vi "MCLB_IndexArray_Tests.vi"(11 "error in":errorcluster) -> (15 "error out":errorcluster)   [LabVIEW 2016, in "DronaTest.lvlib"]
uses:
  DronaTest.lvlib
  APIs/Stimulus/ControlValue/SetValueAuto.vi
  APIs/Stimulus/ControlValue/Controls/MC Listbox/SetValueByArrayIndex.vi
  APIs/Assert/AssertControlValue/Equal.vi
  <vilib>/addons/_JKI Toolkits/Caraya/classes/Assert/Assert Error.vi
  <vilib>/addons/_JKI Toolkits/Caraya/classes/Test/Test.lvclass
  Drona.lvlib
  <vilib>/SLL Toolkit/SLL Debug/SLL Debug.lvlib
  APIs/Stimulus/ControlValue/ControlValue.lvlib
  APIs/Assert/AssertControlValue/AssertControlValue.lvlib
  <vilib>/addons/_JKI Toolkits/Caraya/classes/Assert/Assert.lvclass
  APIs/Stimulus/ControlValue/Controls/MC Listbox/StimulusMCListbox.lvlib
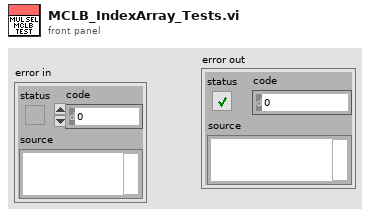
[diagram p1: front panel]
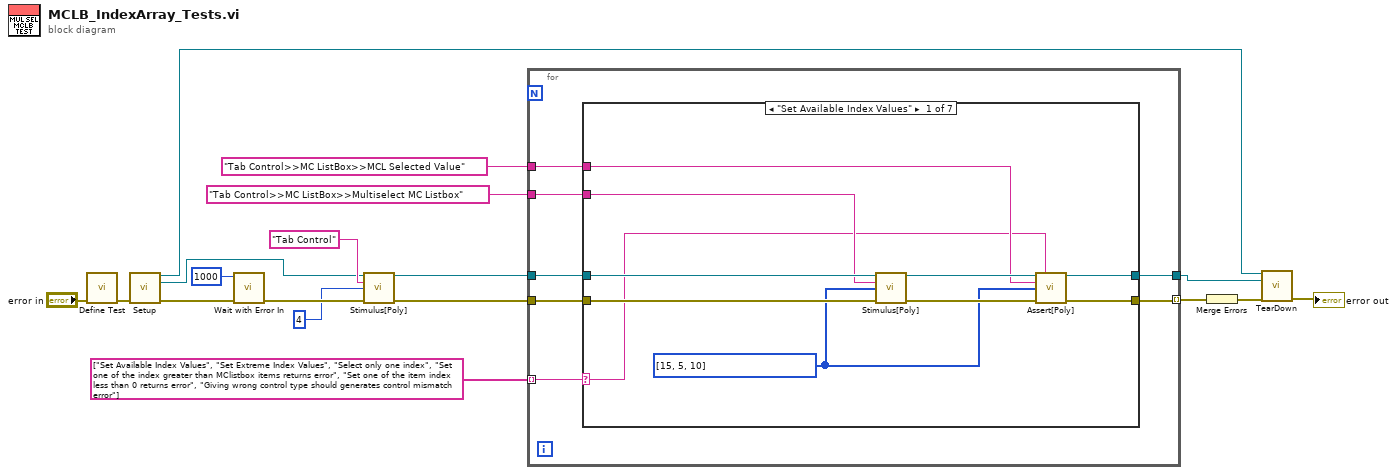
[diagram p0: block diagram]
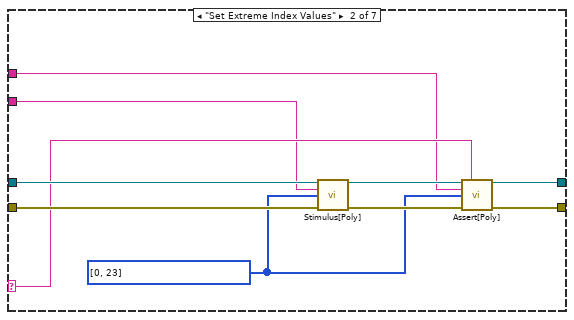
[diagram p2: hidden frame]
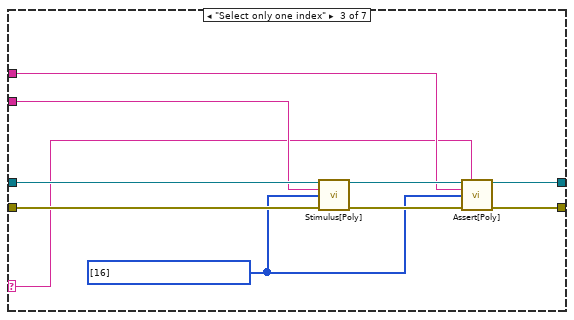
[diagram p3: hidden frame]
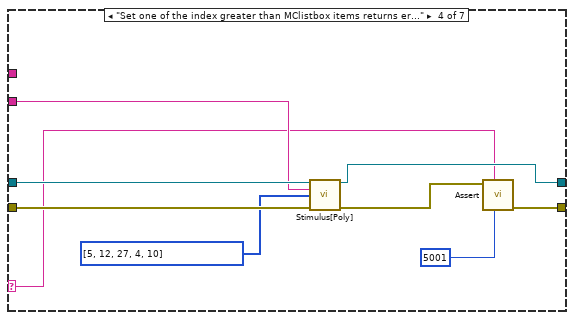
[diagram p4: hidden frame]
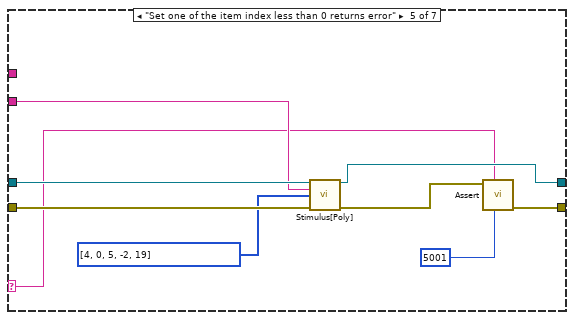
[diagram p5: hidden frame]
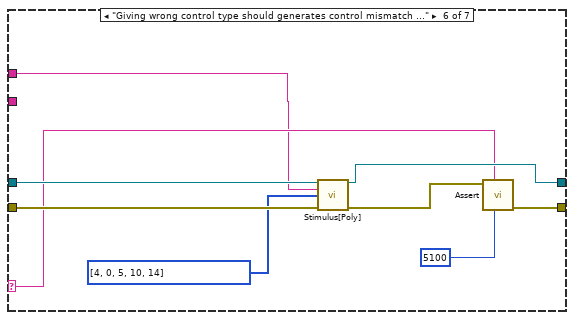
[diagram p6: hidden frame]
diagram:
  n1 = call <vilib>:"Define Test.vi"("error in (no error)"="error in") -> ("error out"=w7:errorcluster)  [unwired: 10 in]
  n2 = call "Setup.vi"("error in (no error)"=w7) -> ("Application Ref"=w2:refnum<vi>, "VI out"=w6:refnum<vi>, "error out"=w5:errorcluster)  [unwired: 12 in]
  n3 = call <vilib>:"Wait with Error In.vi"("error in (no error)"=w5, "milliseconds to wait"=u32 1000) -> ("error out"=w16:errorcluster)  [unwired: 9 in]
  n4 = call-poly "Stimulus[Poly].vi"("VI Reference In"=w6, "Control Path"="Tab Control", "Value (Signaling)"=4, "error in"=w16) -> ("VI Reference Out"=w12:refnum<vi>, "error out"=w15:errorcluster)  [unwired: 10 in]
  n5 = for {
    tunnel: w15 -> [w25]
    tunnel: w12 -> [w24]
    tunnel: "Tab Control>>MC ListBox>>Multiselect MC Listbox" ("Control Path") -> [w23]
    tunnel: "Tab Control>>MC ListBox>>MCL Selected Value" ("Control Path") -> [w22]
    tunnel: [w21] -> w9 mode=indexing
    tunnel: [w20] -> w3
    tunnel: string[] ["Set Available Index Values", "Set Extreme Index Values", "Select only one index", "Set one of the index greater than MClistbox items returns error", "Set one of the item index less than 0 returns error", "Giving wrong control type should generates control mismatch error"] -> [w19] mode=indexing
    n6 = case shown="\"Set Available Index Values\"" w19 {
      selector: w19 -> [w26 w38 w46 w58 w67 w77 _]
      tunnel: w25 -> [w35 w45 w55 w64 w73 w82 w84]
      tunnel: w24 -> [w34 w44 w54 w63 w72 w81 w83]
      tunnel: w23 -> [w33 w36 w53 w62 w71 _ _]
      tunnel: w22 -> [w30 w37 w50 _ _ w74 _]
      tunnel: [w28 w40 w48 w60 w69 w79 w84] -> w21
      tunnel: [w27 w39 w47 w59 w68 w78 w83] -> w20
      frame "Set Available Index Values" {
        w29 = i32[] [15, 5, 10] ("Index Array")
        n7 = call-poly "Stimulus[Poly].vi"("VI Reference In"=w34, "Control Path"=w33, "Index Array"=w29, "Error In"=w35) -> ("VI Reference Out"=w31:refnum<vi>, "Error Out"=w32:errorcluster)  [unwired: 10 in]
        n8 = call-poly "Assert[Poly].vi"("VI Reference In"=w31, "Test Label"=w26, "Control Path"=w30, "Control Value"=w29, "Error In"=w32) -> ("VI Reference Out"=w27:refnum<vi>, "Error Out"=w28:errorcluster)  [unwired: 8 in, 1 out]
      }
      frame "Set Extreme Index Values" {
        w41 = i32[] [0, 23] ("Index Array")
        n9 = call-poly "Stimulus[Poly].vi"("VI Reference In"=w44, "Control Path"=w36, "Index Array"=w41, "Error In"=w45) -> ("VI Reference Out"=w42:refnum<vi>, "Error Out"=w43:errorcluster)  [unwired: 10 in]
        n10 = call-poly "Assert[Poly].vi"("VI Reference In"=w42, "Test Label"=w38, "Control Path"=w37, "Control Value"=w41, "Error In"=w43) -> ("VI Reference Out"=w39:refnum<vi>, "Error Out"=w40:errorcluster)  [unwired: 8 in, 1 out]
      }
      frame "Select only one index" {
        w49 = i32[] [16] ("Index Array")
        n11 = call-poly "Stimulus[Poly].vi"("VI Reference In"=w54, "Control Path"=w53, "Index Array"=w49, "Error In"=w55) -> ("VI Reference Out"=w51:refnum<vi>, "Error Out"=w52:errorcluster)  [unwired: 10 in]
        n12 = call-poly "Assert[Poly].vi"("VI Reference In"=w51, "Test Label"=w46, "Control Path"=w50, "Control Value"=w49, "Error In"=w52) -> ("VI Reference Out"=w47:refnum<vi>, "Error Out"=w48:errorcluster)  [unwired: 8 in, 1 out]
      }
      frame "Set one of the index greater than MClistbox items returns error" {
        n13 = call-poly "Stimulus[Poly].vi"("VI Reference In"=w63, "Control Path"=w62, "Index Array"=i32[] [5, 12, 27, 4, 10], "Error In"=w64) -> ("VI Reference Out"=w59:refnum<vi>, "Error Out"=w57:errorcluster)  [unwired: 10 in]
        n14 = call-poly <vilib>:"Assert.vi"("error code (1)"=5001, "Label"=w58, "Error?"=w57) -> ("error out"=w60:errorcluster)  [unwired: 8 in]
      }
      frame "Set one of the item index less than 0 returns error" {
        n15 = call-poly "Stimulus[Poly].vi"("VI Reference In"=w72, "Control Path"=w71, "Index Array"=i32[] [4, 0, 5, -2, 19], "Error In"=w73) -> ("VI Reference Out"=w68:refnum<vi>, "Error Out"=w66:errorcluster)  [unwired: 10 in]
        n16 = call-poly <vilib>:"Assert.vi"("error code (1)"=5001, "Label"=w67, "Error?"=w66) -> ("error out"=w69:errorcluster)  [unwired: 8 in]
      }
      frame "Giving wrong control type should generates control mismatch error" {
        n17 = call-poly "Stimulus[Poly].vi"("VI Reference In"=w81, "Control Path"=w74, "Index Array"=i32[] [4, 0, 5, 10, 14], "Error In"=w82) -> ("VI Reference Out"=w78:refnum<vi>, "Error Out"=w76:errorcluster)  [unwired: 10 in]
        n18 = call-poly <vilib>:"Assert.vi"("error code (1)"=5100, "Label"=w77, "Error?"=w76) -> ("error out"=w79:errorcluster)  [unwired: 8 in]
      }
      frame Default {
      }
    }
  }
  n19 = Merge Errors(w9) -> (w4:errorcluster)
  n20 = call "TearDown.vi"("Application Ref"=w2, "VI in"=w3, "error in (no error)"=w4) -> ("error out"=→"error out":errorcluster)  [unwired: 12 in]
